vi "NI6071E.StopDAQ.vi"(0 "i ref in":refnum<vi>, 4 "timeout ms (60000)":i32=60000, 5 "error in (no error)":errorcluster) -> (14 "i ref out":refnum<vi>, 19 "error out":errorcluster)   [LabVIEW 2014, in "NI6071E.lvlib"]
uses:
  NI6071E.lvlib
  NI6071ECommandCluster.ctl
  NI6071ECommand.ctl
panel:
  in  "PPMA Command":T1=enum."ConfigureDAQ"
  in  "PPMA Command Cluster":T2
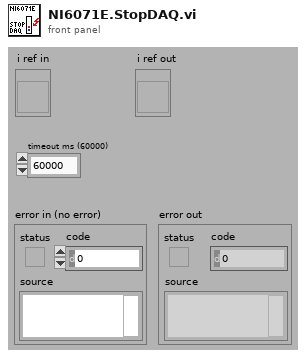
[diagram p1: front panel]
types:
  T1 = typedef "NI6071E.lvlib/NI6071ECommand.ctl" = enum16{"Ping", "Reset", "ConfigureDAQ", "StartDAQ", "StopDAQ", "GetDAQStatus", "ReadData", "SaveData", "CloseConnection"}
  T2 = typedef "NI6071E.lvlib/NI6071ECommandCluster.ctl" = cluster{"Command":string, "Data":string, "error out":errorcluster}
  T3 = typedef "NI6071E.lvlib/NI6071E.i attribute.ctl" = cluster{"NI6071E Server":string, "Port":u16, "NI6071E Config":T4, "NI6071E Start":T5, "Waveforms":waveform(dbl)[], "RT Error":errorcluster, "NI6071E Read":T6, "connection ID":refnum<k5>, "DAQ Status":string, "device (1)":i16, "DAQ Status Service ID":i32}
  T4 = typedef "NI6071E.lvlib/NI6071EConfig.ctl" = cluster{"device (1)":i16, "channels (0)":tag[], "buffer size (1000 scans)":i32, "[number of buffers] (1)":i32, "measurement mode structure":cluster{"measurement mode":u16, "reserved":u32}, "input limits (no change)":cluster{"high limit (0.0)":sgl, "low limit (0.0)":sgl}[], "coupling & input config (no change:0)":cluster{"coupling (no change:0)":enum16{"no change", "DC", "AC", "GND", "internal ref."}, "input config (no change:0)":u16}[]}
  T5 = typedef "NI6071E.lvlib/NI6071EStart.ctl" = cluster{"scan rate (40000 scans/sec)":sgl, "trigger type (analog)":enum16{"no trigger", "analog", "digital A", "digital A & B", "scan clock gate"}, "edge or slope \n(rising)":enum16{"no change", "rising", "falling"}, "number of buffers to acquire (1)":i32, "analog chan (PFI0) & level (2.00)":cluster{"trigger channel (empty)":string, "level (0.0)":sgl}, "[additional trig params]":cluster{"hysteresis (0.0)":sgl, "coupling (no change:0)":enum16{"no change", "DC", "AC"}, "delay (0 sec)":sgl, "skip count (0)":i32, "time limit (0 sec)":sgl}}
  T6 = typedef "NI6071E.lvlib/NI6071ERead.ctl" = cluster{"time limit in sec (-1:auto calculate)":sgl, "number of scans to read (-1:all)":i32}
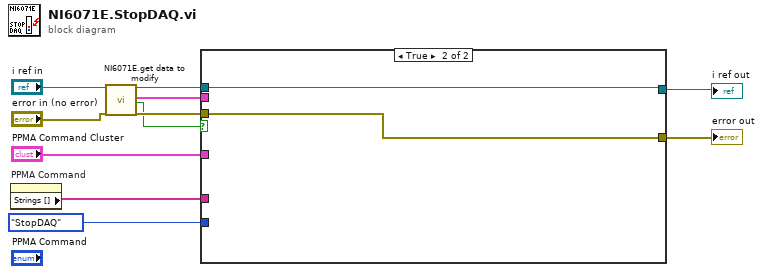
[diagram p0: block diagram]
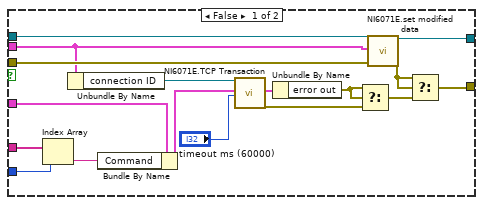
[diagram p2: hidden frame]
diagram:
  n1 = property on="PPMA Command" class="Enum (strict)"() -> ("Strings []"=w4:string[])  [unwired: 2 in, 2 out]
  n2 = call "NI6071E.get data to modify.vi"("i ref in"="i ref in", "error in (no error)"="error in (no error)") -> ("i ref out"=w8:refnum<vi>, "i attribute"=w2:T3, "timed out"=w1:bool, "error out"=w9:errorcluster)  [unwired: 14 in]
  n3 = case shown="True" w1 {
    tunnel: w9 -> [w28 w29]
    tunnel: w8 -> [w27 w30]
    tunnel: [w26 w30] -> w7
    tunnel: [w24 w29] -> w6
    tunnel: "PPMA Command Cluster" -> [w22 _]
    tunnel: w4 -> [w20 _]
    tunnel: NI6071ECommand."StopDAQ" ("PPMA Command") -> [w19 _]
    tunnel: w2 -> [w12 _]
    frame False {
      n4 = Index Array(array=w20, index=w19) -> (element=w18:string)
      n5 = Unbundle By Name(w12) -> ("connection ID"=w23:refnum<k5>)
      n6 = Bundle By Name(cluster=w22, "Command"=w18) -> (w21:T2)
      n7 = call "NI6071E.TCP Transaction.vi"("connection ID in"=w23, "NI6071E Command Cluster"=w21, "timeout ms (25000)"="timeout ms (60000)") -> ("NI6071E Response"=w16:T2, "error out"=w14:errorcluster)  [unwired: 14 in, 1 out]
      n8 = Unbundle By Name(w16) -> ("error out"=w15:errorcluster)
      n9 = Select(t=w15, s=w15, f=w14) -> (s? t:f=w13:errorcluster)
      n10 = call "NI6071E.set modified data.vi"("i ref in"=w27, "i attribute"=w12, "error in (no error)"=w28) -> ("i ref out"=w26:refnum<vi>, "error out"=w25:errorcluster)  [unwired: 15 in]
      n11 = Select(t=w25, s=w25, f=w13) -> (s? t:f=w24:errorcluster)
    }
    frame True {
    }
  }
  "i ref out" <- w7
  "error out" <- w6
